vi "CalcTimerPeroid.vi"(6 "Exclude Inputs?":bool, 11 "TimePeroid":i32[](array[numeric])) -> (3 "Proper TimePeroid":i32)   [LabVIEW 2017, in "TimerEngine.lvlib" / "TimerEngine.lvclass"]
uses:
  TimerEngine.lvclass
  <userlib>/_OpenG.lib/array/array.llb/Remove Duplicates from 1D Array (I32)__ogtk.vi
  <userlib>/_OpenG.lib/array/array.llb/Filter 1D Array (I32)__ogtk.vi
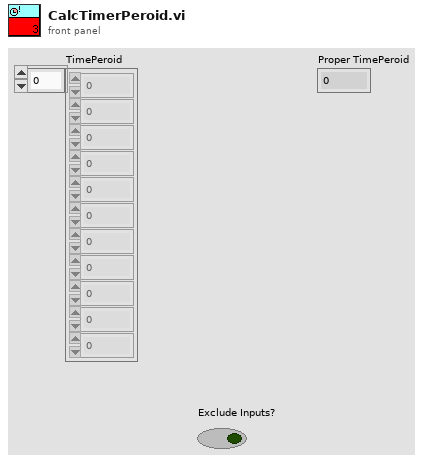
[diagram p1: front panel]
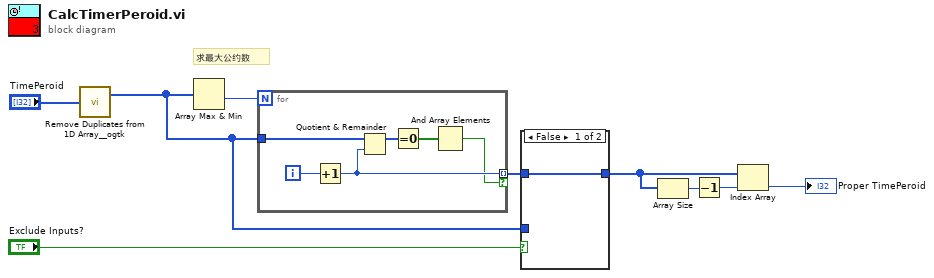
[diagram p0: block diagram]
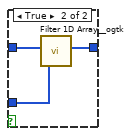
[diagram p2: hidden frame]
diagram:
  # "求最大公约数"
  n1 = call-poly <userlib>:"Remove Duplicates from 1D Array__ogtk.vi"("Input Array"="TimePeroid") -> ("Output Array"=w1:i32[])  [unwired: 1 out]
  n2 = Array Max & Min(array=w1) -> (min value=w5:i32)  [unwired: 3 out]
  n3 = for {
    N: w5 -> [_]
    tunnel: [w11] -> w7 mode=indexing if=w10
    tunnel: w1 -> [w13]
    i -> [w14]
    n4 = Increment(x=w14) -> (x+1=w11:i32)
    n5 = Quotient & Remainder(x=w13, y=w11) -> (x-y*floor(x/y)=w15:i32[])  [unwired: 1 out]
    n6 = Equal To 0?(x=w15) -> (x = 0?=w12:bool[])
    n7 = And Array Elements(Boolean array=w12) -> (logical AND=w10:bool)
  }
  n8 = case shown="False" "Exclude Inputs?" {
    tunnel: w7 -> [w16 w19]
    tunnel: [w16 w18] -> w6
    tunnel: w1 -> [_ w17]
    frame False {
    }
    frame True {
      n9 = call-poly <userlib>:"Filter 1D Array__ogtk.vi"("items to filter"=w17, "array"=w19) -> ("filtered array"=w18:i32[])  [unwired: 4 in, 1 out]
    }
  }
  n10 = Array Size(array=w6) -> (size(s)=w9:i32)
  n11 = Decrement(x=w9) -> (x-1=w8:i32)
  n12 = Index Array(array=w6, index=w8) -> (element=→"Proper TimePeroid":i32)
